vi "niDTS WLAN Dut Rx Configure.vi"(0 "Dut Handle in":T6, 5 "niDTS WLAN DUT Parameters":T1={"WLAN Type"=enum."n - MCS7", "Bandwidth (Hz)"=enum."20 MHz", "Channel"=36, "Guard Interval"=enum."SHORT", "FEC Coding"=enum."LDPC", "Power (dBm)"=0.0, "Payload Length (bytes)"=1500, "16 Symbols"=TRUE, "Chains"=[TRUE, FALSE, FALSE, FALSE]}, 7 "Apply Additional Defaults":bool=TRUE, 11 "error in (no error)":errorcluster) -> (4 "Dut Handle":T6, 15 "error out":errorcluster)   [LabVIEW 2015, in "niDTS WLAN.lvlib"]
doc: "Set the basic parameters for the WLAN TX Test. \n\nInputs:\n* Apply Additional Defaults. This allows more advanced parameters, which are dependant on the inputs, to have their default values set.\n\nCallbacks:\n* WLAN DUT Additional Defaults\n\nNote: This behavior is expected to be depricated when full parameter sets are passed as inputs and the input dependant defaults are calculated on the top parameter setting level."
uses:
  niDTS WLAN.lvlib
  Framework/Dut/Includes/niDTS Dut INC Handle.ctl
  Framework/Dut/Objects/BASE_class/niDTS Dut.lvclass
  Includes/niDTS WLAN DUT INC Parameters.ctl
  Includes/niDTS WLAN INC Type.ctl
  Includes/niDTS WLAN INC CH BW.ctl
  Includes/niDTS WLAN INC GI.ctl
  Includes/niDTS WLAN INC FEC Coding.ctl
  Includes/niDTS WLAN Dut INC Handle.ctl
  Objects/BASE_class/niDTS WLAN Dut.lvclass
  Objects/niDTS WLAN Dut Data/niDTS WLAN Dut Data.lvclass
  Framework/Logger/Objects/BASE_class/niDTS Logger.lvclass
  Framework/niDTS Framework.lvlib
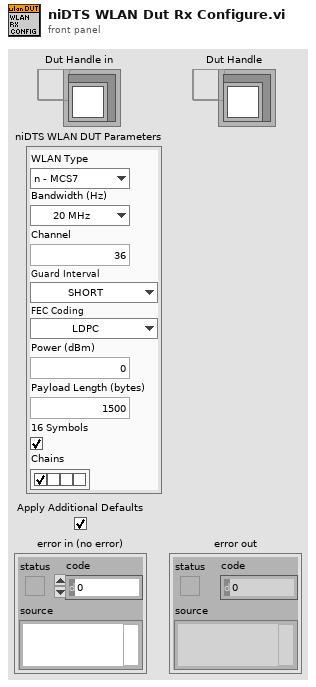
[diagram p1: front panel]
types:
  T1 = typedef "niDTS WLAN.lvlib/niDTS WLAN DUT INC Parameters.ctl" = cluster{"WLAN Type":T2, "Bandwidth (Hz)":T3, "Channel":i32, "Guard Interval":T4, "FEC Coding":T5, "Power (dBm)":dbl, "Payload Length (bytes)":i32, "16 Symbols":bool, "Chains":bool[]}
  T2 = typedef "niDTS WLAN.lvlib/niDTS WLAN INC Type.ctl" = enum16{"b - 1 Mbps", "b - 2 Mbps", "b - 5.5 Mbps", "b - 11 Mbps", "ag - 6 Mbps", "ag - 9 Mbps", "ag - 12 Mbps", "ag - 18 Mbps", "ag - 24 Mbps", "ag - 36 Mbps", "ag - 48 Mbps", "ag - 54 Mbps", "n - MCS0", "n - MCS1", "n - MCS2", "n - MCS3", "n - MCS4", "n - MCS5", "n - MCS6", "n - MCS7", "n - MCS8", "n - MCS9", "n - MCS10", "n - MCS11", "n - MCS12", "n - MCS13", "n - MCS14", "n - MCS15", "n - MCS16", "n - MCS17", "n - MCS18", "n - MCS19", "n - MCS20", "n - MCS21", "n - MCS22", "n - MCS23", "n - MCS24", "n - MCS25", "n - MCS26", "n - MCS27", "n - MCS28", "n - MCS29", "n - MCS30", "n - MCS31", "ac - MCS0 -1", "ac - MCS1 -1", "ac - MCS2 -1", "ac - MCS3 -1", "ac - MCS4 -1", "ac - MCS5 -1", "ac - MCS6 -1", "ac - MCS7 -1", "ac - MCS8 -1", "ac - MCS9 -1", "ac - MCS0 -2", "ac - MCS1 -2", "ac - MCS2 -2", "ac - MCS3 -2", "ac - MCS4 -2", "ac - MCS5 -2", "ac - MCS6 -2", "ac - MCS7 -2", "ac - MCS8 -2", "ac - MCS9 -2", "ac - MCS0 -3", "ac - MCS1 -3", "ac - MCS2 -3", "ac - MCS3 -3", "ac - MCS4 -3", "ac - MCS5 -3", "ac - MCS6 -3", "ac - MCS7 -3", "ac - MCS8 -3", "ac - MCS9 -3", "ac - MCS0 -4", "ac - MCS1 -4", "ac - MCS2 -4", "ac - MCS3 -4", "ac - MCS4 -4", "ac - MCS5 -4", "ac - MCS6 -4", "ac - MCS7 -4", "ac - MCS8 -4", "ac - MCS9 -4"}
  T3 = typedef "niDTS WLAN.lvlib/niDTS WLAN INC CH BW.ctl" = enum16{"20 MHz", "40 MHz", "80 MHz", "160 MHz"}
  T4 = typedef "niDTS WLAN.lvlib/niDTS WLAN INC GI.ctl" = enum16{"LONG", "SHORT"}
  T5 = typedef "niDTS WLAN.lvlib/niDTS WLAN INC FEC Coding.ctl" = enum16{"BCC", "LDPC"}
  T6 = typedef "niDTS Framework.lvlib/niDTS Dut INC Handle.ctl" = refnum<data-value>
  T7 = typedef "niDTS WLAN.lvlib/niDTS WLAN Dut INC Handle.ctl" = refnum<data-value>
  T8 = typedef "niDTS Framework.lvlib/niDTS Logger INC Handle.ctl" = refnum<data-value>
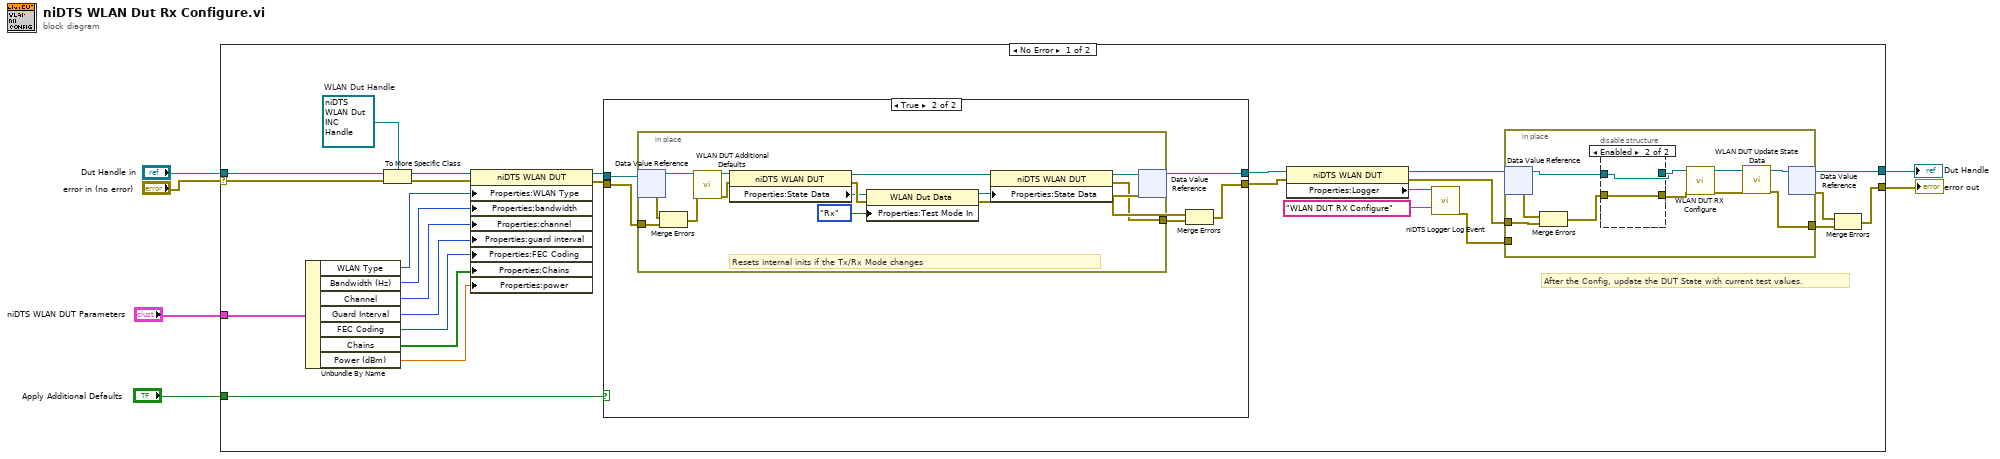
[diagram p0: block diagram]
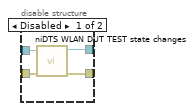
[diagram p2: hidden frame]
diagram:
  n1 = case shown="No Error" "error in (no error)" {
    selector: "error in (no error)" -> [w21 w72]
    tunnel: "Dut Handle in" -> [w33 w73]
    tunnel: "niDTS WLAN DUT Parameters" -> [w29 _]
    tunnel: "Apply Additional Defaults" -> [w24 _]
    tunnel: [w20 w73] -> w3
    tunnel: [w17 w72] -> w2
    frame No Error {
      w32 = T7 refnum  # WLAN Dut Handle
      # "After the Config, update the DUT State with current test values."
      n2 = Unbundle By Name(w29) -> ("WLAN Type"=w28:T2, "Bandwidth (Hz)"=w8:T3, "Channel"=w27:i32, "Guard Interval"=w26:T4, "FEC Coding"=w7:T5, "Chains"=w25:bool[], "Power (dBm)"=w16:dbl)
      n3 = To More Specific Class(target class=w32, reference=w33, error in=w21) -> (specific class reference=w31:T7, error out=w30:errorcluster)
      n4 = property class="niDTS WLAN DUT"(reference=w31, error in=w30, "Properties:WLAN Type"=w28, "Properties:bandwidth"=w8, "Properties:channel"=w27, "Properties:guard interval"=w26, "Properties:FEC Coding"=w7, "Properties:Chains"=w25, "Properties:power"=w16) -> (reference out=w23:T7, error out=w22:errorcluster)
      n5 = case shown="True" w24 {
        tunnel: w23 -> [w51 w57]
        tunnel: w22 -> [w50 w56]
        tunnel: [w51 w53] -> w15
        tunnel: [w50 w52] -> w14
        frame False {
        }
        frame True {
          n6 = in-place {
            in-place-border: [w58] -> w55
            in-place-border: w56 -> [w70]
            # "Resets internal inits if the Tx/Rx Mode changes"
            n7 = in-place-dvr #1(w57) -> (w71:refnum<class "niDTS WLAN Dut.lvclass">, w69:errorcluster)
            n8 = Merge Errors(w69, w70) -> (w68:errorcluster)
            n9 = call-dynamic "WLAN DUT Additional Defaults.vi"("niDTS WLAN DUT in"=w71, "error in (no error)"=w68) -> ("niDTS WLAN DUT out"=w61:refnum<class "niDTS WLAN Dut.lvclass">, "error out"=w60:errorcluster)  [unwired: 12 in]
            n10 = property class="niDTS WLAN DUT"(reference=w61, error in=w60) -> (reference out=w62:refnum<class "niDTS WLAN Dut.lvclass">, error out=w64:errorcluster, "Properties:State Data"=w63:refnum<class "niDTS WLAN Dut Data.lvclass">)
            n11 = property class="WLAN Dut Data"(reference=w63, error in=w64, "Properties:Test Mode In"=enum16{"Tx", "Rx"}."Rx" ("Test Mode In")) -> (reference out=w66:refnum<class "niDTS WLAN Dut Data.lvclass">, error out=w65:errorcluster)
            n12 = property class="niDTS WLAN DUT"(reference=w62, error in=w65, "Properties:State Data"=w66) -> (reference out=w59:refnum<class "niDTS WLAN Dut.lvclass">, error out=w58:errorcluster)
            n13 = in-place-dvr #1(w59) -> (w53:T7, w54:errorcluster)
          }
          n14 = Merge Errors(w54, w55) -> (w52:errorcluster)
        }
      }
      n15 = property class="niDTS WLAN DUT"(reference=w15, error in=w14) -> (reference out=w11:T7, error out=w10:errorcluster, "Properties:Logger"=w13:T8)
      n16 = call "niDTS Logger Log Event.vi"("Logger Handle"=w13, "Source/Location"="WLAN DUT RX Configure") -> ("error out"=w9:errorcluster)  [unwired: 11 in, 2 out]
      n17 = in-place {
        in-place-border: w10 -> [w43]
        in-place-border: [w38] -> w19
        in-place-border: w9 -> [_]
        n18 = in-place-dvr #2(w11) -> (w36:refnum<class "niDTS WLAN Dut.lvclass">, w42:errorcluster)
        n19 = Merge Errors(w42, w43) -> (w37:errorcluster)
        n20 = disable-structure shown="Enabled" {
          disable-tunnel: w36 -> [w47 w49]
          disable-tunnel: [w46 w49] -> w35
          disable-tunnel: w37 -> [w45 w48]
          disable-tunnel: [w44 w48] -> w34
          frame Disabled {
            n21 = call-dynamic "niDTS WLAN DUT TEST state changes.vi"("error in (no error)"=w45, "niDTS WLAN DUT in"=w47) -> ("error out"=w44:errorcluster, "niDTS WLAN DUT out"=w46:refnum<class "niDTS WLAN Dut.lvclass">)  [unwired: 8 in]
          }
          frame Enabled {
          }
        }
        n22 = call-dynamic "WLAN DUT RX Configure.vi"("niDTS WLAN DUT in"=w35, "error in (no error)"=w34) -> ("niDTS WLAN DUT out"=w41:refnum<class "niDTS WLAN Dut.lvclass">, "error out"=w39:errorcluster)  [unwired: 12 in]
        n23 = call-dynamic "WLAN DUT Update State Data.vi"("error in (no error)"=w39, "niDTS WLAN DUT in"=w41) -> ("error out"=w38:errorcluster, "niDTS WLAN DUT out"=w40:refnum<class "niDTS WLAN Dut.lvclass">)  [unwired: 8 in]
        n24 = in-place-dvr #2(w40) -> (w20:T7, w18:errorcluster)
      }
      n25 = Merge Errors(w18, w19) -> (w17:errorcluster)
    }
    frame Error {
    }
  }
  "error out" <- w2
  "Dut Handle" <- w3
